vi "Prepare Test Naming.vi"(8 "error in":errorcluster, 11 "Report Generator in":refnum<class "Report Generator.lvclass">) -> (0 "error out":errorcluster, 3 "Report Generator out":refnum<class "Report Generator.lvclass">)   [LabVIEW 2023, in "Report Generator.lvlib" / "Report Generator.lvclass"]
uses:
  Library/Report Generator.lvclass
  Library/Report Generator.lvclass/Report Generator.ctl
  builds/Tools/Report.lvlibp/Accessors/Write UUT_Name.vi
  builds/Tools/Report.lvlibp/Accessors/Write Test Name.vi
  builds/Tools/Report.lvlibp/Accessors/Write Tester.vi
  builds/Tools/Report.lvlibp/Accessors/Write Witness.vi
  builds/Tools/Report.lvlibp/Report.lvclass
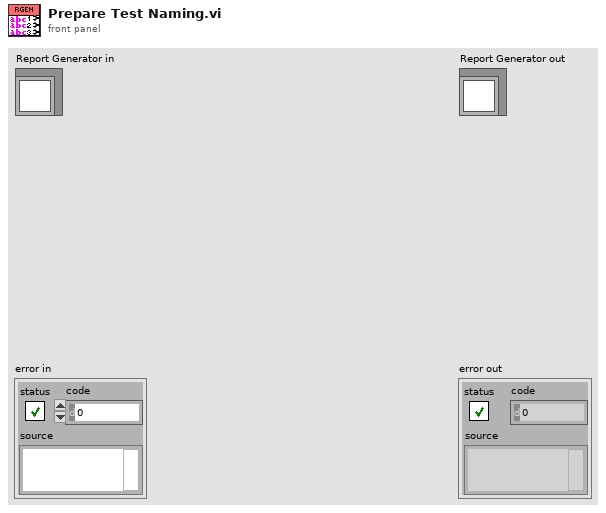
[diagram p1: front panel]
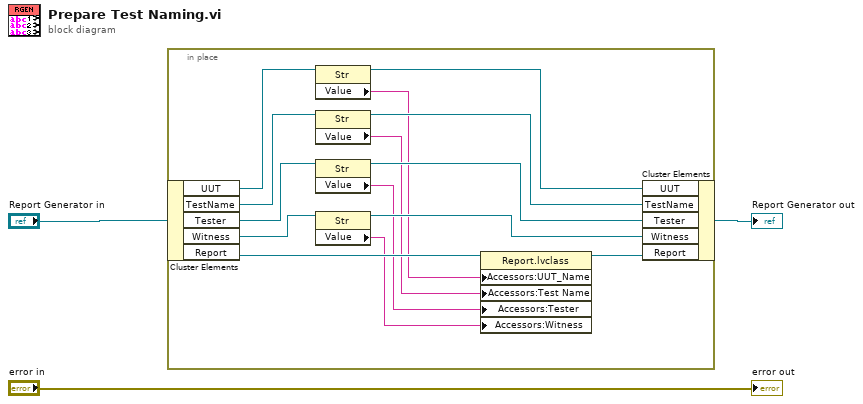
[diagram p0: block diagram]
diagram:
  n1 = in-place {
    n2 = in-place-cluster #1("Report Generator in") -> ("UUT"=w15:refnum<vi>, "TestName"=w14:refnum<vi>, "Tester"=w13:refnum<vi>, "Witness"=w12:refnum<vi>, "Report"=w17:refnum<class "Report.lvclass">)
    n3 = property class="Str"(reference=w15) -> (reference out=w8:refnum<vi>, "Value"=w4:string)  [unwired: 1 in, 1 out]
    n4 = property class="Str"(reference=w14) -> (reference out=w9:refnum<vi>, "Value"=w5:string)  [unwired: 1 in, 1 out]
    n5 = property class="Str"(reference=w13) -> (reference out=w10:refnum<vi>, "Value"=w6:string)  [unwired: 1 in, 1 out]
    n6 = property class="Str"(reference=w12) -> (reference out=w11:refnum<vi>, "Value"=w7:string)  [unwired: 1 in, 1 out]
    n7 = property class="Report.lvclass"(reference=w17, "Accessors:UUT_Name"=w4, "Accessors:Test Name"=w5, "Accessors:Tester"=w6, "Accessors:Witness"=w7) -> (reference out=w16:refnum<class "Report.lvclass">)  [unwired: 1 in, 1 out]
    n8 = in-place-cluster #1("UUT"=w8, "TestName"=w9, "Tester"=w10, "Witness"=w11, "Report"=w16) -> (→"Report Generator out":refnum<class "Report Generator.lvclass">)
  }
  "error out" <- "error in"
